vi "ComputeFontScaleFromRequiredHeight.vi"(6 "Thickness (Default: 1)":i32=1, 7 "OpenCV Font Face":T1, 8 "error in (no error)":errorcluster, 11 "Required Text Height":u16) -> (0 "error out":errorcluster, 3 "Font Scale":dbl)   [LabVIEW 2020, in "g_ar_toolkit.image.lvlib"]
uses:
  g_ar_toolkit.image.lvlib
  Font Face.ctl
  bin/g_ar_toolkit.1.32.dll
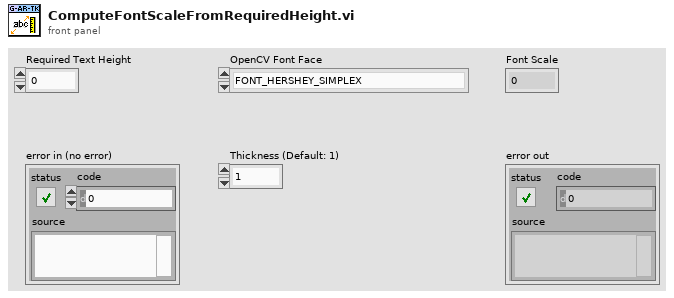
[diagram p1: front panel]
types:
  T1 = typedef "g_ar_toolkit.image.lvlib/Font Face.ctl" = enum16{"FONT_HERSHEY_SIMPLEX", "FONT_HERSHEY_PLAIN", "FONT_HERSHEY_DUPLEX", "FONT_HERSHEY_COMPLEX", "FONT_HERSHEY_TRIPLEX", "FONT_HERSHEY_COMPLEX_SMALL", "FONT_HERSHEY_SCRIPT_SIMPLEX", "FONT_HERSHEY_SCRIPT_COMPLEX", "FONT_ITALIC"}
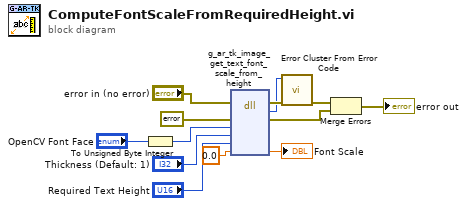
[diagram p0: block diagram]
diagram:
  n1 = To Unsigned Byte Integer(number="OpenCV Font Face") -> (unsigned 8bit integer=w10:u8)
  n2 = dll-call lib="C:/serenial/libraries/g-augmented-reality-toolkit/LabVIEW/bin/g_ar_toolkit.1.*.*" fn="g_ar_tk_image_get_text_font_scale_from_height"(error in="error in (no error)", "error_cluster"=errorcluster {"status"=FALSE, "code"=0, "source"=""} ("error constant"), "font_face"=w10, "thickness"="Thickness (Default: 1)", "Required Height"="Required Text Height", "Font Scale"=0.0) -> (error out=w9:errorcluster, "MgErr"=w8:i32, "error_cluster"=w5:errorcluster, "Font Scale"=→"Font Scale":dbl)  [unwired: 5 in, 1 out]
  n3 = call <vilib>:"Error Cluster From Error Code.vi"("error in (no error)"=w9, "error code (0)"=w8) -> ("error out"=w7:errorcluster)  [unwired: 7 in]
  n4 = Merge Errors(w7, w5) -> (→"error out":errorcluster)
